vi "SNAP.vi"(9 "Take Snap":bool, 10 "stop":bool, 11 "Session Out":T1) -> (3 "Number_of_photos 2":i32)   [LabVIEW 2015]
uses:
  <vilib>/userdefined/High Color/IMAQdx.ctl
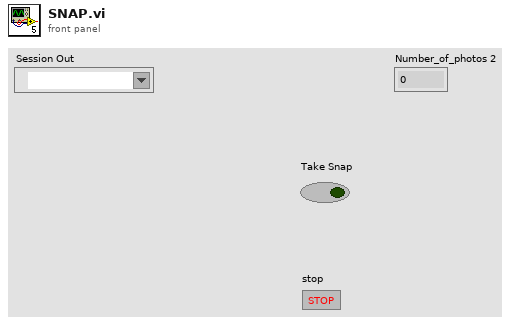
[diagram p1: front panel]
types:
  T1 = typedef "IMAQdx.ctl" = refnum<k21>
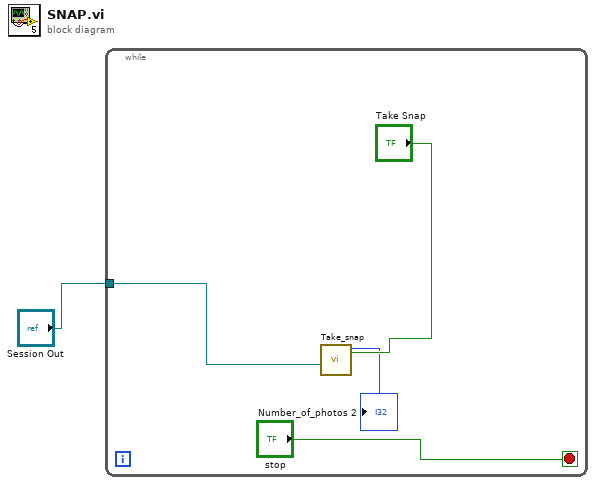
[diagram p0: block diagram]
diagram:
  n1 = while {
    tunnel: "Session Out" -> [w3]
    stop <- "stop" stop-if-true
    n2 = call "Take_snap.vi"("Take_snap"="Take Snap", "Camera Session"=w3) -> ("Number_of_photos 2"=→"Number_of_photos 2":i32)  [unwired: 9 in]
  }
